vi "UTA0504_PWM_Test.vi"() -> ()   [LabVIEW 2010]
panel:
  in  "pConfig":T1={"Prescaler[0]"=240, "Prescaler[1]"=240, "Prescaler[2]"=240, "Prescaler[3]"=240, "Prescaler[4]"=240, "Prescaler[5]"=240, "Prescaler[6]"=240, "Prescaler[7]"=240, "Precision[0]"=1000, "Precision[1]"=1000, "Precision[2]"=1000, "Precision[3]"=1000, "Precision[4]"=1000, "Precision[5]"=1000, "Precision[6]"=1000, "Precision[7]"=1000, "Pulse[0]"=500, "Pulse[1]"=500, "Pulse[2]"=500, "Pulse[3]"=500, "Pulse[4]"=500, "Pulse[5]"=500, "Pulse[6]"=500, "Pulse[7]"=500, "Phase[0]"=0, "Phase[1]"=0, "Phase[2]"=0, "Phase[3]"=0, "Phase[4]"=0, "Phase[5]"=0, "Phase[6]"=0, "Phase[7]"=0, "Polarity[0]"=0, "Polarity[1]"=0, "Polarity[2]"=0, "Polarity[3]"=0, "Polarity[4]"=0, "Polarity[5]"=0, "Polarity[6]"=0, "Polarity[7]"=0, "ChannelMask"=192} {"ChannelMask" format="%x"}
  in  "ChannelMask":u8=63 format="%x"
  in  "Device Index":i32(ring) items=["0", "1", "2", "3", "4", "5"]
  # "PWM_CH0-->LIN1"
  # "PWM_CH1-->LIN2"
  # "PWM_CH2-->LIN3"
  # "PWM_CH3->LIN4"
  # "PWM_CH4-->DO0"
  # "PWM_CH5->DO1"
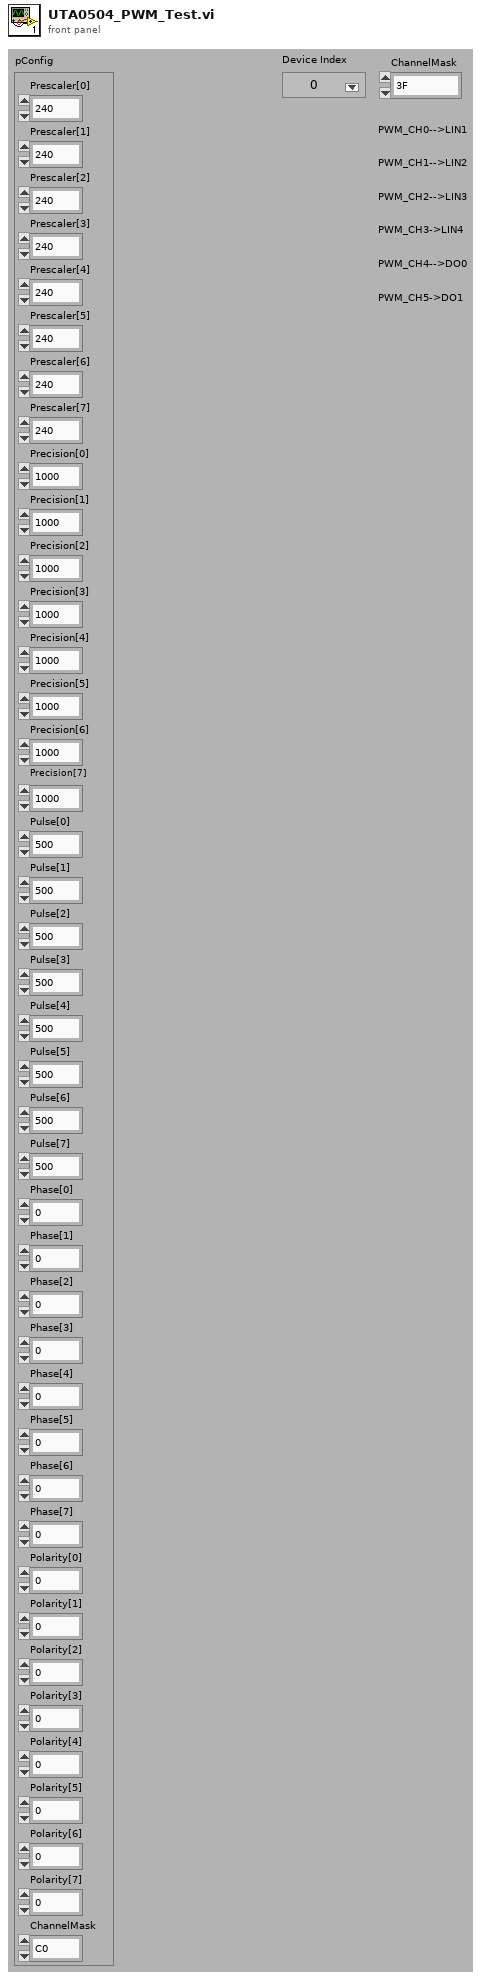
[diagram p1: front panel]
types:
  T1 = cluster{"Prescaler[0]":u16, "Prescaler[1]":u16, "Prescaler[2]":u16, "Prescaler[3]":u16, "Prescaler[4]":u16, "Prescaler[5]":u16, "Prescaler[6]":u16, "Prescaler[7]":u16, "Precision[0]":u16, "Precision[1]":u16, "Precision[2]":u16, "Precision[3]":u16, "Precision[4]":u16, "Precision[5]":u16, "Precision[6]":u16, "Precision[7]":u16, "Pulse[0]":u16, "Pulse[1]":u16, "Pulse[2]":u16, "Pulse[3]":u16, "Pulse[4]":u16, "Pulse[5]":u16, "Pulse[6]":u16, "Pulse[7]":u16, "Phase[0]":u16, "Phase[1]":u16, "Phase[2]":u16, "Phase[3]":u16, "Phase[4]":u16, "Phase[5]":u16, "Phase[6]":u16, "Phase[7]":u16, "Polarity[0]":u8, "Polarity[1]":u8, "Polarity[2]":u8, "Polarity[3]":u8, "Polarity[4]":u8, "Polarity[5]":u8, "Polarity[6]":u8, "Polarity[7]":u8, "ChannelMask":u8}
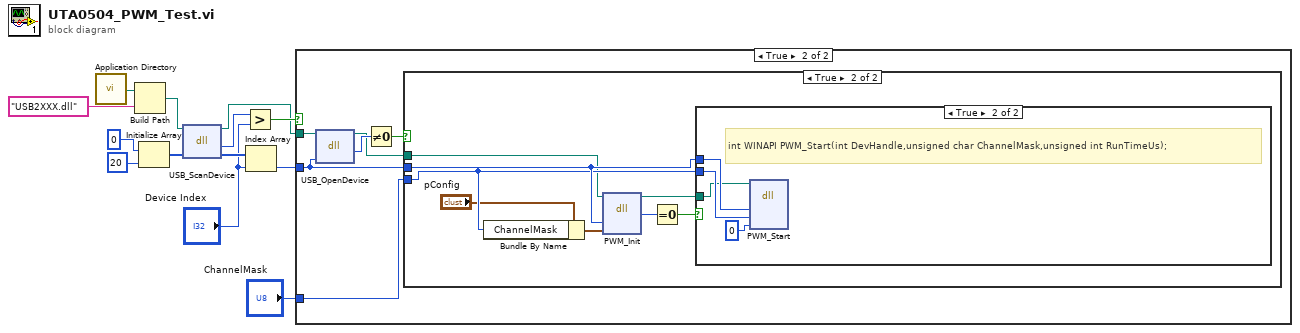
[diagram p0: block diagram]
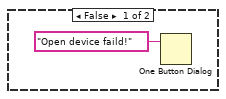
[diagram p3: hidden frame]
diagram:
  n1 = call <vilib>:"Application Directory.vi"() -> ("Application Directory"=w3:path)
  n2 = Build Path(base path=w3, name or relative path="USB2XXX.dll") -> (appended path=w2:path)
  n3 = Initialize Array(0, 20 ("dimension size")) -> (w10:i32[])
  n4 = dll-call lib="E:/Projects/USB2XXX_Example/sdk/api/Labview/USB2XXX.*" fn="USB_ScanDevice"(path in=w2, "pDevNum"=w10) -> (path out=w1:path, "return type"=w9:i32, "pDevNum"=w13:i32[])  [unwired: 2 in, 1 out]
  n5 = Greater?(x=w9, y="Device Index") -> (0:w7:bool)
  n6 = Index Array(array=w13, index="Device Index") -> (element=w6:i32)
  n7 = case shown="True" w7 {
    tunnel: w6 -> [_ w16]
    tunnel: "ChannelMask" -> [_ w17]
    tunnel: w1 -> [_ w15]
    frame False {
    }
    frame True {
      n8 = dll-call lib="E:/Projects/USB2XXX_Example/sdk/api/Labview/USB2XXX.*" fn="USB_OpenDevice"(path in=w15, "DevIndex"=w16) -> (path out=w14:path, "return type"=w19:u8)  [unwired: 3 in, 1 out]
      n9 = Not Equal To 0?(x=w19) -> (x != 0?=w18:bool)
      n10 = case shown="True" w18 {
        tunnel: w17 -> [_ w24]
        tunnel: w16 -> [_ w25]
        tunnel: w14 -> [_ w22]
        frame False {
          n11 = One Button Dialog(message="Open device faild!") -> ()  [unwired: 1 in, 1 out]
        }
        frame True {
          n12 = Bundle By Name(cluster="pConfig", "ChannelMask"=w24) -> (w28:T1)
          n13 = dll-call lib="E:/Projects/USB2XXX_Example/sdk/api/Labview/USB2XXX.dll" fn="PWM_Init"(path in=w22, "DevHandle"=w25, "pConfig"=w28) -> (path out=w21:path, "return type"=w27:i32)  [unwired: 4 in, 1 out]
          n14 = Equal To 0?(x=w27) -> (x = 0?=w26:bool)
          n15 = case shown="True" w26 {
            tunnel: w25 -> [_ w31]
            tunnel: w24 -> [_ w30]
            tunnel: w21 -> [_ w29]
            frame False {
            }
            frame True {
              # "int WINAPI PWM_Start(int DevHandle,unsigned char ChannelMask,unsigned int RunTimeUs);"
              n16 = dll-call lib="E:/Projects/USB2XXX_Example/sdk/api/Labview/USB2XXX.dll" fn="PWM_Start"(path in=w29, "DevHandle"=w31, "ChannelMask"=w30, "RunTimeUs"=u32 0) -> ()  [unwired: 6 in, 2 out]
            }
          }
        }
      }
    }
  }
